vi "Get Content Length.vi"(8 "error in (no error)":errorcluster, 10 "header":string) -> (0 "error out":errorcluster, 2 "content length":i32)   [LabVIEW 2020]
uses:
  <vilib>/regexp/Match Regular Expression.xnode
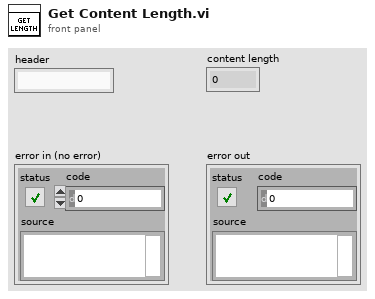
[diagram p1: front panel]
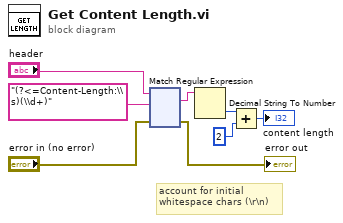
[diagram p0: block diagram]
diagram:
  # "account for initial \nwhitespace chars (\\r\\n)"
  n1 = xnode "Match Regular Expression"("input string"="header", "regular expression"="(?<=Content-Length:\\s)(\\d+)", "error in"="error in (no error)") -> ("whole match"=w1:string, "error out"=→"error out":errorcluster)  [unwired: 3 in, 3 out]
  n2 = Decimal String To Number(string=w1) -> (number=w6:i32)  [unwired: 2 in, 1 out]
  n3 = Add(x=w6, y=2) -> (x+y=→"content length":i32)
